vi "Publish Client Updates.vi"(8 "error in (no error)":errorcluster, 10 "Client Info Loop Data":T1, 11 "TCPMessaging in":refnum<class "TCPMessaging.lvclass">) -> (0 "error out":errorcluster, 3 "TCPMessaging out":refnum<class "TCPMessaging.lvclass">)   [LabVIEW 2020, in "Vecto.lvlib" / "TCPMessaging.lvclass"]
uses:
  TCPMessaging.lvclass
  proto/TcpClientHello/Data.ctl
  proto/TcpClientHello/TcpClientHello.lvlib
  Client Info.ctl
  Vecto.lvlib
  Connected Client.ctl
  Client Info Loop Data.ctl
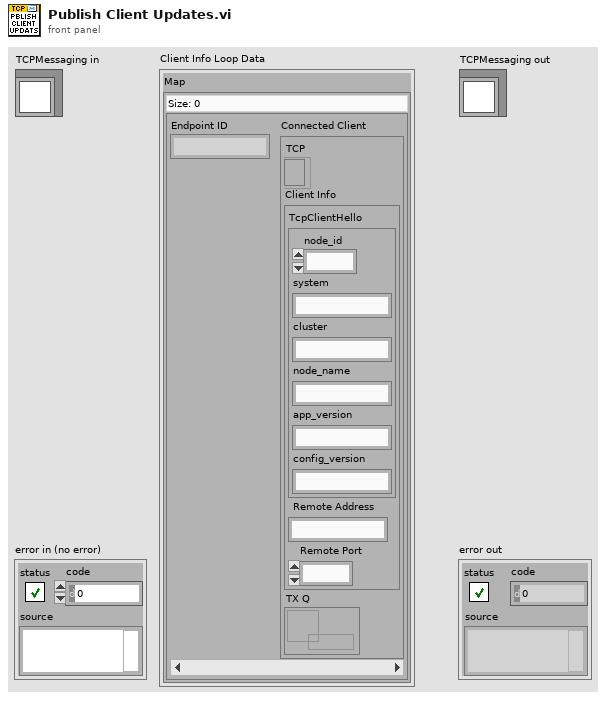
[diagram p1: front panel]
types:
  T1 = typedef "Vecto.lvlib/TCPMessaging.lvclass/Client Info Loop Data.ctl" = cluster{"Map":map{string, T2}}
  T2 = typedef "Vecto.lvlib/TCPMessaging.lvclass/Connected Client.ctl" = cluster{"TCP":refnum<k5>, "Client Info":T3, "TX Q":refnum<queue>}
  T3 = typedef "Vecto.lvlib/Client Info.ctl" = cluster{"TcpClientHello":T4, "Remote Address":string, "Remote Port":u16}
  T4 = typedef "TcpClientHello.lvlib/Data.ctl" = cluster{"node_id":u32, "system":string, "cluster":string, "node_name":string, "app_version":string, "config_version":string}
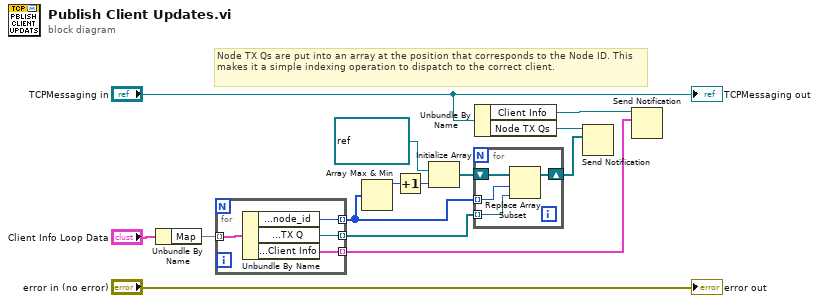
[diagram p0: block diagram]
diagram:
  # "Node TX Qs are put into an array at the position that corresponds to the Node ID. This makes it a simple indexing operation to dispatch to the correct client."
  n1 = Unbundle By Name("Client Info Loop Data") -> ("Map"=w12:map{string, T2})
  n2 = for {
    tunnel: w12 -> [w18] mode=indexing
    tunnel: [w17] -> w3 mode=indexing
    tunnel: [w16] -> w1 mode=indexing
    tunnel: [w15] -> w8 mode=indexing
    n3 = Unbundle By Name(w18) -> ("Connected Client.Client Info.TcpClientHello.node_id"=w16:u32, "Connected Client.TX Q"=w15:refnum<queue>, "Connected Client.Client Info"=w17:T3)
  }
  n4 = Array Max & Min(array=w1) -> (max value=w11:u32)  [unwired: 3 out]
  n5 = Increment(x=w11) -> (x+1=w10:u32)
  n6 = Initialize Array(refnum<queue> refnum ("TX Q"), w10) -> (w7:refnum<queue>[])
  n7 = for {
    tunnel: w8 -> [w19] mode=indexing
    shift-right: [w21] -> w5
    shift-left: w7 -> [w22]
    tunnel: w1 -> [w20] mode=indexing
    n8 = Replace Array Subset(array=w22, new element=w19, index=w20) -> (w21:refnum<queue>[])
  }
  n9 = Unbundle By Name("TCPMessaging in") -> ("Client Info"=w4:refnum<notifier>, "Node TX Qs"=w6:refnum<notifier>)
  n10 = Send Notification(notification=w5, notifier=w6) -> ()  [unwired: 1 in, 2 out]
  n11 = Send Notification(notification=w3, notifier=w4) -> ()  [unwired: 1 in, 2 out]
  "error out" <- "error in (no error)"
  "TCPMessaging out" <- "TCPMessaging in"
